vi "Pockels Cal_Update.vi"(10 "New cal section":string[][](array[string]), 11 "Existing pockels Cal file path":path) -> (2 "Cal file strings":string[][](array[string]), 3 "Create new":bool)   [LabVIEW 2013]
uses:
  Program Files (x86)/National Instruments/LabVIEW 2013/user.lib/My Palettes.lib/Files & paths/Spreadsheet/Read From Spreadsheet File (string)-Mod.vi
  gl_Calibration globals.vi
panel:
  out "New cal section":string[][](array[string])
  out "Loaded cal file":string[][](array[string])
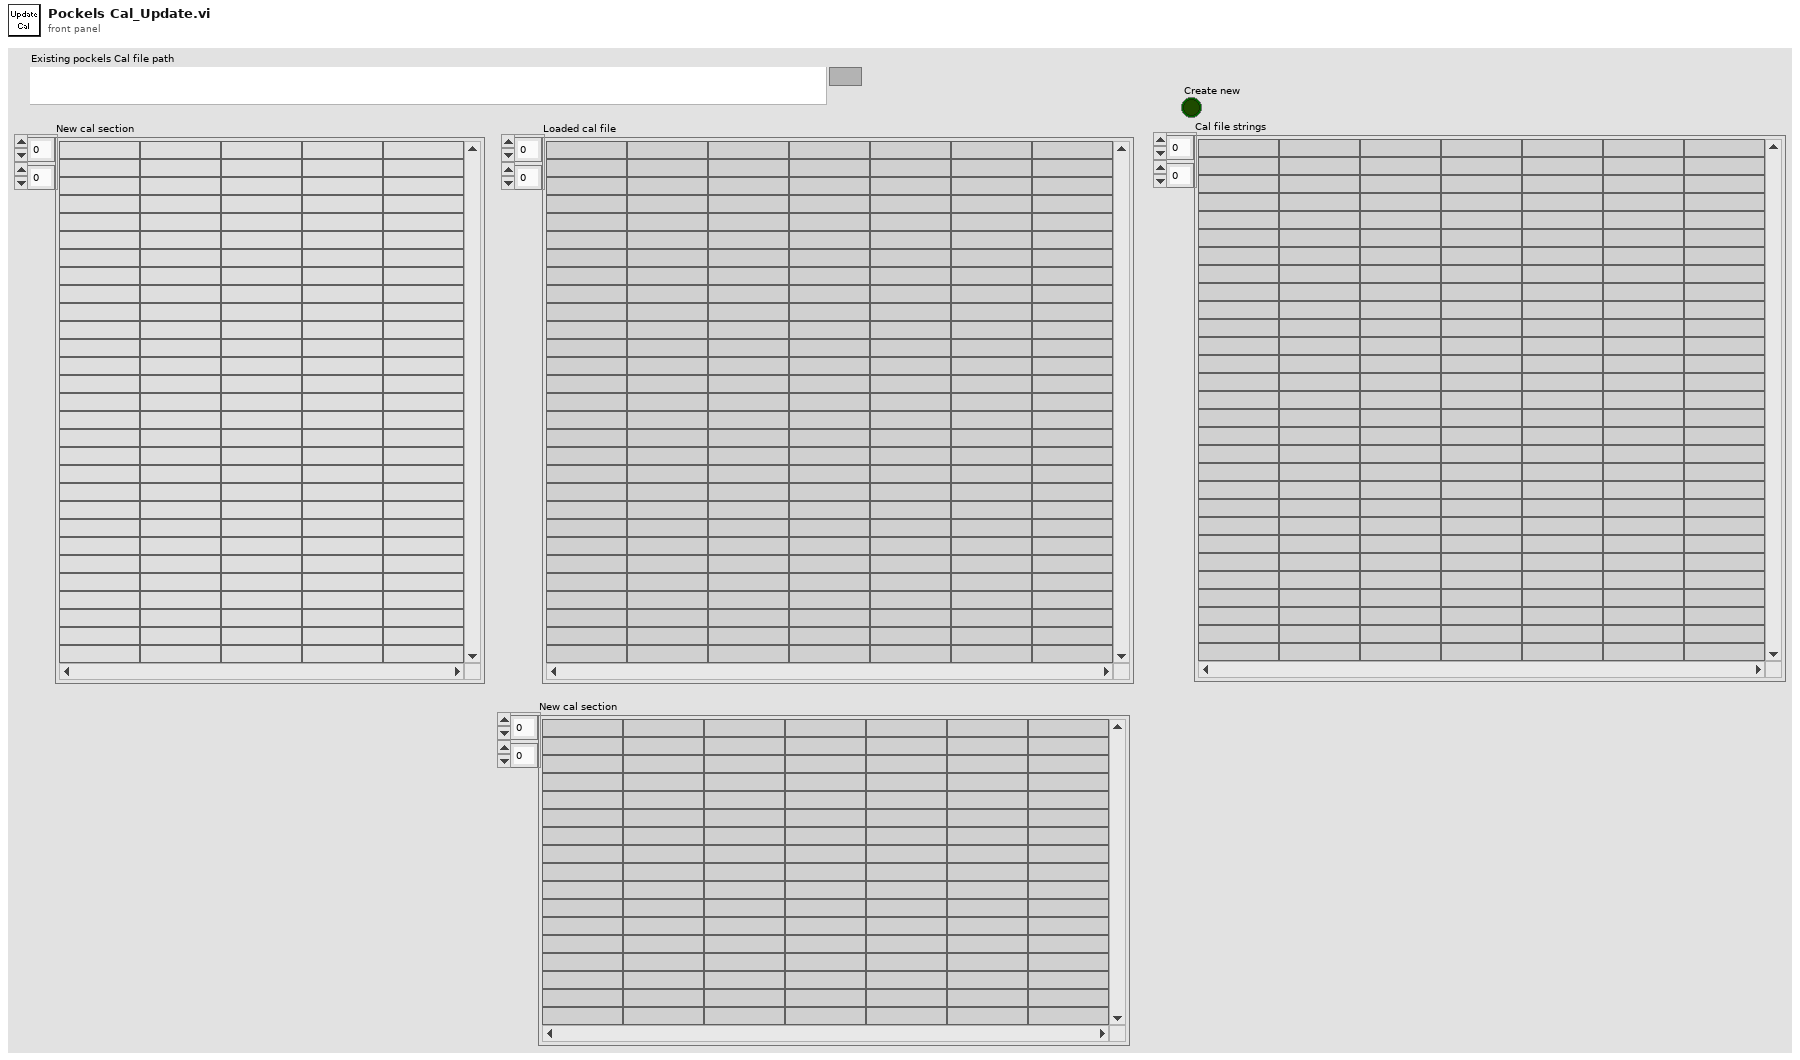
[diagram p1: front panel]
types:
  T1 = typedef "Pockels cal conditions cluster.ctl" = cluster{"Wavelength":u16, "Zoom":u8, "Dwell time (us)":dbl, "Pockels bias":i16, "Prism 1":u16, "Prism 2":u16, "Laser power during pockels cal (mW)":u16}
  T2 = cluster{"Zoom":u8, "Dwell time (us)":dbl, "Pockels bias":i16}
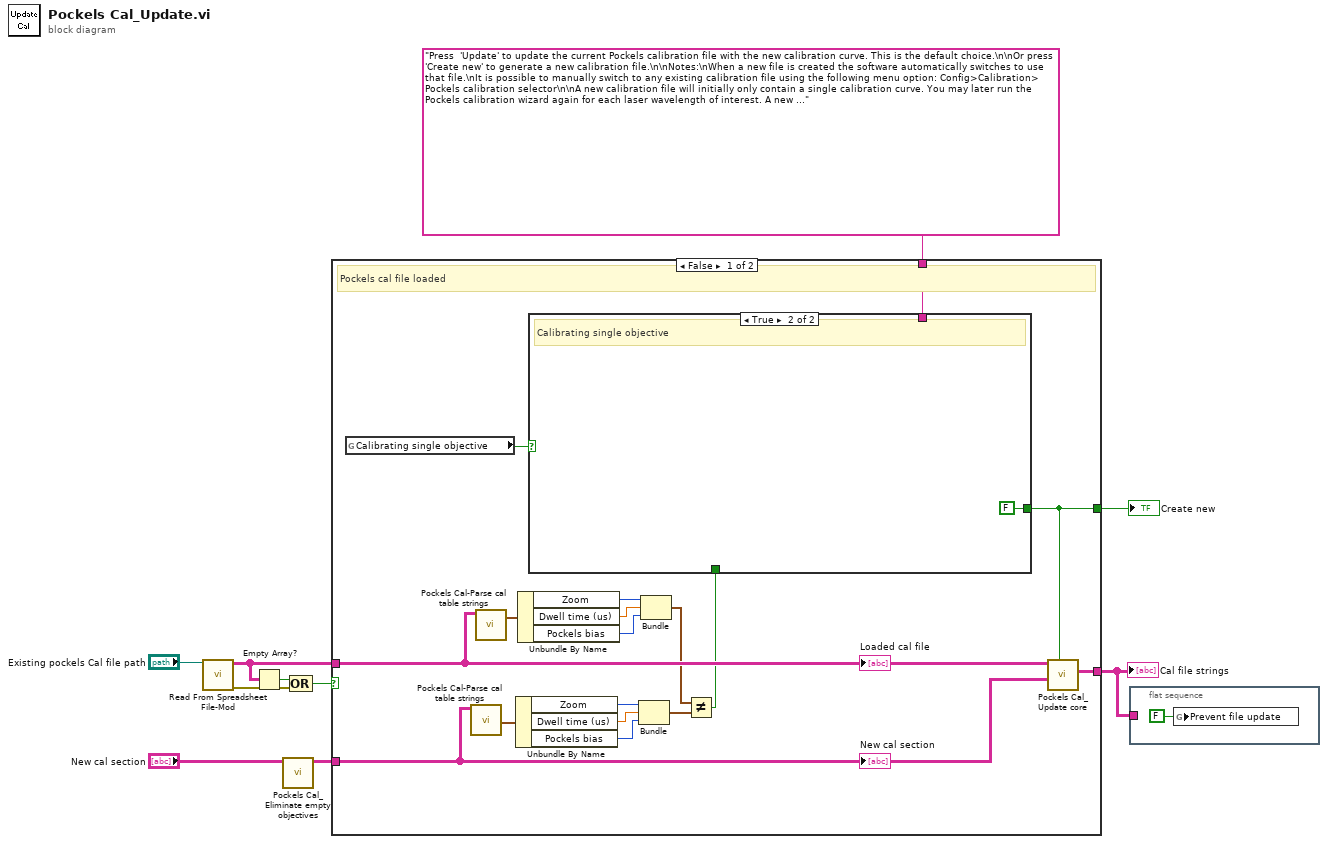
[diagram p0: block diagram]
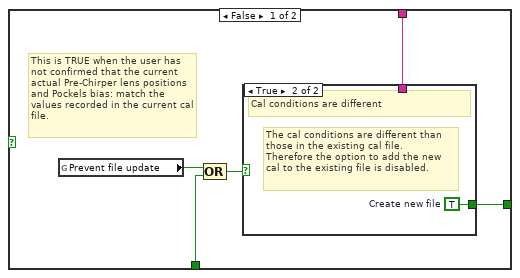
[diagram p2: hidden frame]
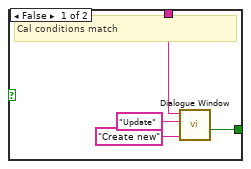
[diagram p3: hidden frame]
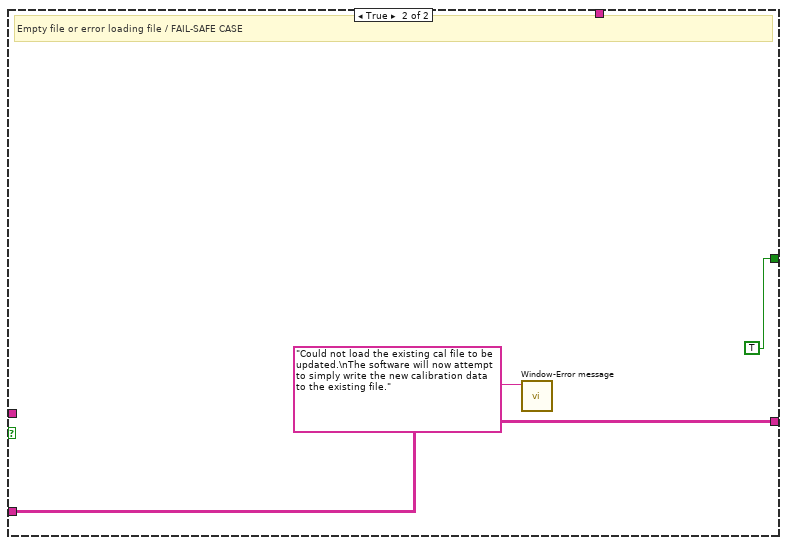
[diagram p4: hidden frame]
diagram:
  n1 = call-poly "Read From Spreadsheet File-Mod.vi"("file path (dialog if empty)"="Existing pockels Cal file path") -> ("all rows"=w7:string[][], "error out"=w9:errorcluster)  [unwired: 9 in, 4 out]
  n2 = Empty Array?(array=w7) -> (empty?=w10:bool)
  n3 = call "Pockels Cal_Eliminate empty objectives.vi"("New cal section"="New cal section") -> ("New cal section"=w3:string[][])  [unwired: 10 in]
  n4 = Compound Arithmetic op=OR(w10, w9) -> (w8:bool)
  n5 = case shown="False" w8 {
    tunnel: w3 -> [w26 w41]
    tunnel: [w27 w41] -> w2
    tunnel: w7 -> [w25 _]
    tunnel: [w15 TRUE] -> w5
    tunnel: "Press  'Update' to update the current Pockels calibration file with the new calibration curve. This is the default choice.\n\nOr press 'Create new' to generate a new calibration file.\n\nNotes:\nWhen a new file is created the software automatically switches to use that file.\nIt is possible to manually switch to any existing calibration file using the following menu option: Config>Calibration> Pockels calibration selector\n\nA new calibration file will initially only contain a single calibration curve. You may later run the Pockels calibration wizard again for each laser wavelength of interest. A new calibration curve will be added each time.\nNew calibration curves may only be added to an existing file if during calibration a set of conditions are still identical to the conditions at the time the file was initially created.\nThe conditions are:\na) Dwell time\nb) Zoom\nc) Pockels bias\n" ("Message string") -> [w14 _]
    frame False {
      # "Pockels cal file loaded"
      n6 = global read "gl_Calibration globals.vi" "Calibrating single objective"() -> (w11:bool)
      n7 = call "Pockels Cal-Parse cal table strings.vi"("SINGLE CAL SET (inc. headers & info)"=w26) -> ("Cal conditions"=w24:T1)  [unwired: 5 in, 5 out]
      n8 = call "Pockels Cal-Parse cal table strings.vi"("SINGLE CAL SET (inc. headers & info)"=w25) -> ("Cal conditions"=w20:T1)  [unwired: 5 in, 5 out]
      n9 = Unbundle By Name(w24) -> ("Zoom"=w23:u8, "Dwell time (us)"=w22:dbl, "Pockels bias"=w12:i16)
      n10 = Unbundle By Name(w20) -> ("Zoom"=w21:u8, "Dwell time (us)"=w19:dbl, "Pockels bias"=w13:i16)
      n11 = Bundle("Zoom"=w23, "Dwell time (us)"=w22, "Pockels bias"=w12) -> (w17:T2)  [unwired: 1 in]
      n12 = Bundle("Zoom"=w21, "Dwell time (us)"=w19, "Pockels bias"=w13) -> (w18:T2)  [unwired: 1 in]
      n13 = Not Equal?(x=w18, y=w17) -> (x != y?=w16:bool)
      n14 = case shown="True" w11 {
        tunnel: w16 -> [w31 _]
        tunnel: [w29 FALSE ("Create new file")] -> w15
        tunnel: w14 -> [w28 _]
        frame False {
          # "This is TRUE when the user has not confirmed that the current actual Pre-Chirper lens positions and Pockels bias: match the values recorded in the current cal file."
          n15 = global read "gl_Calibration globals.vi" "Prevent file update"() -> (w30:bool)
          n16 = Compound Arithmetic op=OR(w30, w31) -> (w32:bool)
          n17 = case shown="True" w32 {
            tunnel: [w34 w37] -> w29
            tunnel: w28 -> [w33 _]
            frame False {
              # "Cal conditions match"
              n18 = call "Dialogue Window.vi"("Caption-Left button (Cancel)"="Create new", "Caption-Right button (OK)"="Update", "Message string"=w33) -> ("Cancelled (Left button pressed)"=w34:bool)  [unwired: 6 in, 2 out]
            }
            frame True {
              w37 = TRUE  # Create new file
              # "The cal conditions are different than those in the existing cal file.\nTherefore the option to add the new cal to the existing file is disabled."
              # "Cal conditions are different"
            }
          }
        }
        frame True {
          # "Calibrating single objective"
        }
      }
      n19 = call "Pockels Cal_Update core.vi"("Create new?"=w15, "New cal section (empty objectives removed)"=w26, "Loaded cal file"=w25) -> ("Cal file strings"=w27:string[][])  [unwired: 8 in]
      "Loaded cal file" <- w25
      "New cal section" <- w26
    }
    frame True {
      # "Empty file or error loading file / FAIL-SAFE CASE"
      n20 = call "Window-Error message.vi"("Message"="Could not load the existing cal file to be updated.\nThe software will now attempt to simply write the new calibration data to the existing file.") -> ()  [unwired: 10 in, 1 out]
    }
  }
  "Cal file strings" <- w2
  "Create new" <- w5
  n21 = flat-sequence {
    tunnel: w2 -> [_]
    frame #0 {
      n22 = global write "gl_Calibration globals.vi" "Prevent file update"(FALSE ("Prevent file update")) -> ()
    }
  }
